vi "Host_Relocation.vi"() -> ()   [LabVIEW 2014]
uses:
  <vilib>/Instr/_visa.llb/VISA Configure Serial Port (Instr).vi
panel:
  out "ERROut?":string
  out "RoughZPrePos":dbl
  in  "Move Forward":bool
  in  "Move Backward":bool
  in  "StepLen um":dbl format="%#_13g"
  in  "MoveTo":bool
  in  "MoveToPos mm":dbl format="%#_13g"
  in  "Confirm":bool
  out "RoughZInitPos mm":dbl
  out "RoughZPosDia":dbl(graph)
  in  "RoughZ":refnum<visa-resource-name>
  out "ERRIn?":string
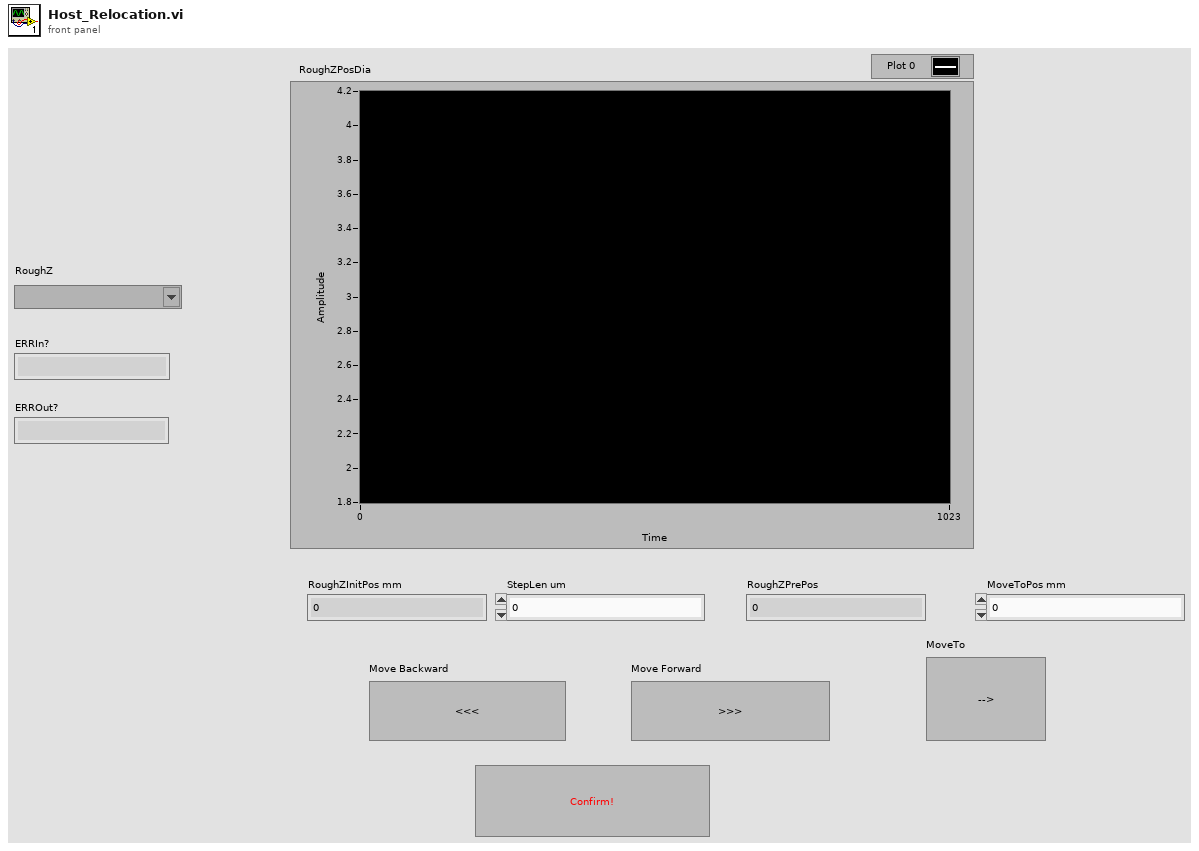
[diagram p1: front panel]
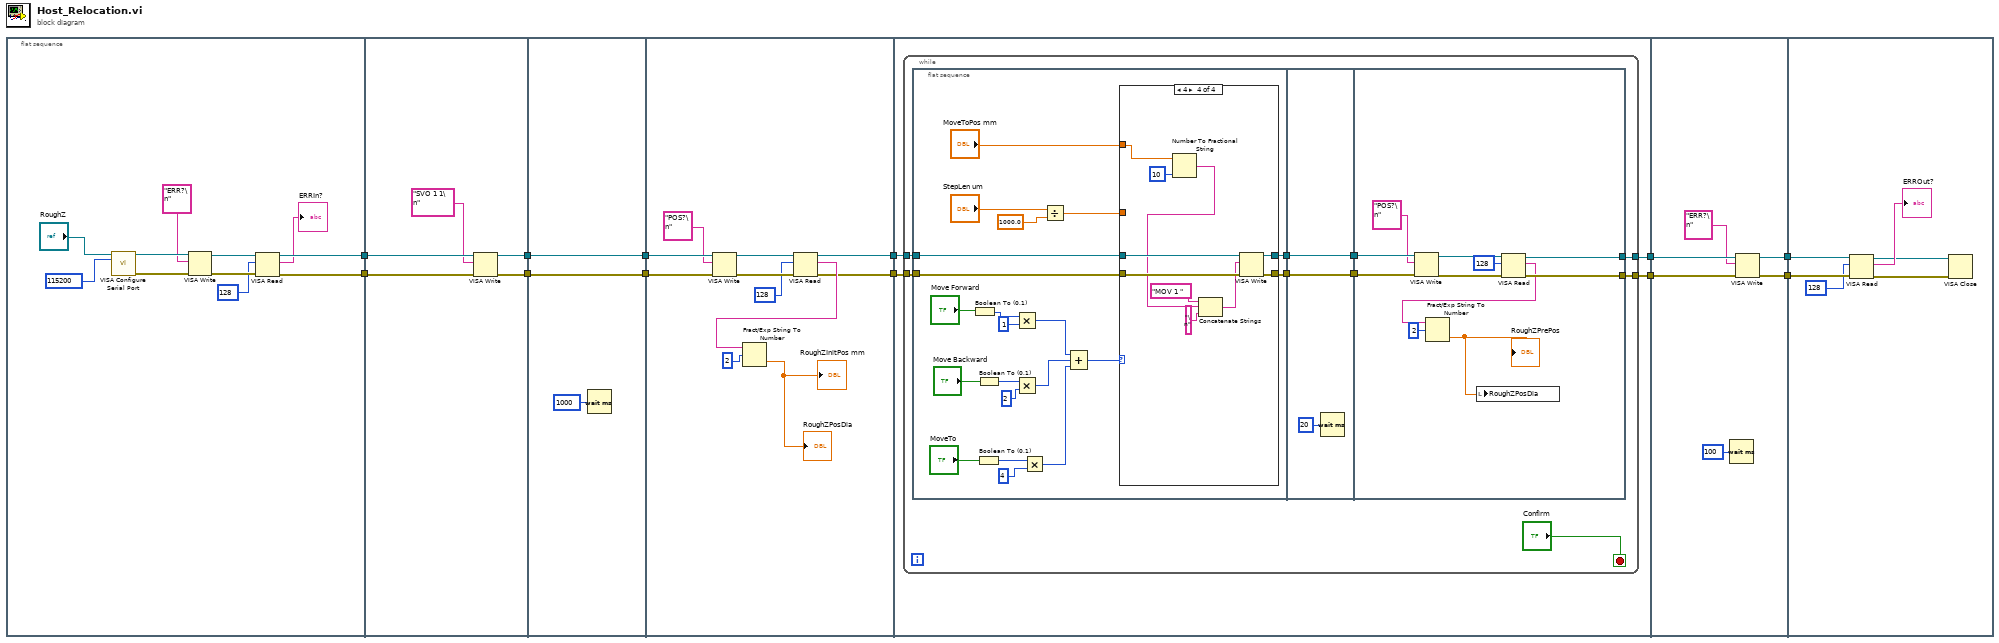
[diagram p0: block diagram]
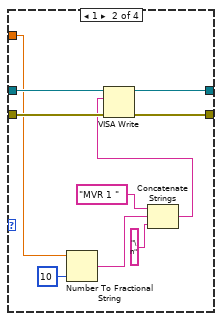
[diagram p3: hidden frame]
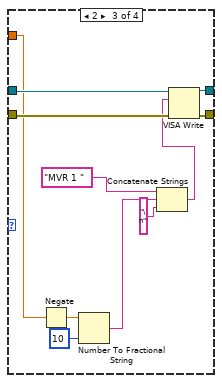
[diagram p4: hidden frame]
diagram:
  n1 = flat-sequence {
    tunnel: [w17] -> w12
    tunnel: [w16] -> w11
    tunnel: w12 -> [w28]
    tunnel: w11 -> [w27]
    tunnel: [w25] -> w10
    tunnel: [w24] -> w9
    tunnel: w10 -> [w30]
    tunnel: w9 -> [w29]
    tunnel: [w30] -> w8
    tunnel: [w29] -> w7
    tunnel: w8 -> [w42]
    tunnel: w7 -> [w41]
    tunnel: [w34] -> w6
    tunnel: [w33] -> w5
    tunnel: w6 -> [w46]
    tunnel: w5 -> [w45]
    tunnel: [w44] -> w4
    tunnel: [w43] -> w3
    tunnel: w4 -> [w128]
    tunnel: w3 -> [w127]
    tunnel: [w125] -> w2
    tunnel: [w124] -> w1
    tunnel: w2 -> [w135]
    tunnel: w1 -> [w134]
    frame #0 {
      n2 = call-poly "VISA Configure Serial Port"("VISA resource name"="RoughZ", "baud rate (9600)"=u32 115200) -> ("VISA resource name out"=w21:refnum<visa-resource-name>, "error out"=w20:errorcluster)  [unwired: 12 in]
      n3 = VISA Write(VISA resource name=w21, write buffer="ERR?\n", error in (no error)=w20) -> (VISA resource name out=w19:refnum<visa-resource-name>, error out=w18:errorcluster)  [unwired: 1 out]
      n4 = VISA Read(VISA resource name=w19, byte count=u32 128, error in (no error)=w18) -> (VISA resource name out=w17:refnum<visa-resource-name>, read buffer=→"ERRIn?":string, error out=w16:errorcluster)  [unwired: 1 out]
    }
    frame #1 {
      n5 = VISA Write(VISA resource name=w28, write buffer="SVO 1 1\n", error in (no error)=w27) -> (VISA resource name out=w25:refnum<visa-resource-name>, error out=w24:errorcluster)  [unwired: 1 out]
    }
    frame #2 {
      n6 = Wait (ms)(milliseconds to wait=u32 1000) -> ()  [unwired: 1 out]
    }
    frame #3 {
      n7 = VISA Write(VISA resource name=w42, write buffer="POS?\n", error in (no error)=w41) -> (VISA resource name out=w39:refnum<visa-resource-name>, error out=w38:errorcluster)  [unwired: 1 out]
      n8 = VISA Read(VISA resource name=w39, byte count=u32 128, error in (no error)=w38) -> (VISA resource name out=w34:refnum<visa-resource-name>, read buffer=w36:string, error out=w33:errorcluster)  [unwired: 1 out]
      n9 = Fract/Exp String To Number(string=w36, offset=2) -> (number=→"RoughZInitPos mm" →"RoughZPosDia":dbl)  [unwired: 2 in, 1 out]
    }
    frame #4 {
      n10 = while {
        tunnel: w46 -> [w54]
        tunnel: w45 -> [w53]
        tunnel: [w48] -> w44
        tunnel: [w47] -> w43
        stop <- "Confirm" stop-if-true
        n11 = flat-sequence {
          tunnel: w54 -> [w67]
          tunnel: w53 -> [w66]
          tunnel: [w65] -> w52
          tunnel: [w64] -> w51
          tunnel: w52 -> [w111]
          tunnel: w51 -> [w110]
          tunnel: [w111] -> w50
          tunnel: [w110] -> w49
          tunnel: w50 -> [w123]
          tunnel: w49 -> [w122]
          tunnel: [w117] -> w48
          tunnel: [w116] -> w47
          frame #0 {
            n12 = Boolean To (0,1)(Boolean="Move Forward") -> (0, 1=w71:i16)
            n13 = Boolean To (0,1)(Boolean="MoveTo") -> (0, 1=w59:i16)
            n14 = Boolean To (0,1)(Boolean="Move Backward") -> (0, 1=w69:i16)
            n15 = Multiply(x=w71, y=i16 1) -> (x*y=w63:i16)
            n16 = Multiply(x=w69, y=i16 2) -> (x*y=w62:i16)
            n17 = Multiply(x=w59, y=i16 4) -> (x*y=w57:i16)
            n18 = Divide(x="StepLen um", y=1000.0) -> (x/y=w74:dbl)
            n19 = Compound Arithmetic op=ADD(w63, w62, w57) -> (w61:i16)
            n20 = case shown="4" w61 {
              tunnel: w74 -> [_ w84 w94 _]
              tunnel: w67 -> [w78 w88 w99 w109]
              tunnel: w66 -> [w77 w87 w98 w108]
              tunnel: [w78 w80 w97 w107] -> w65
              tunnel: [w77 w79 w96 w106] -> w64
              tunnel: "MoveToPos mm" -> [_ _ _ w105]
              frame 0, Default {
              }
              frame 1 {
                n21 = Number To Fractional String(number=w84, precision (6)=i16 10) -> (F-format string=w82:string)  [unwired: 2 in]
                n22 = Concatenate Strings("MVR 1 " ("string"), w82, "\n" ("string")) -> (w86:string)
                n23 = VISA Write(VISA resource name=w88, write buffer=w86, error in (no error)=w87) -> (VISA resource name out=w80:refnum<visa-resource-name>, error out=w79:errorcluster)  [unwired: 1 out]
              }
              frame 2 {
                n24 = Negate(x=w94) -> (-x=w95:dbl)
                n25 = Number To Fractional String(number=w95, precision (6)=i16 10) -> (F-format string=w91:string)  [unwired: 2 in]
                n26 = Concatenate Strings("MVR 1 " ("string"), w91, "\n" ("string")) -> (w89:string)
                n27 = VISA Write(VISA resource name=w99, write buffer=w89, error in (no error)=w98) -> (VISA resource name out=w97:refnum<visa-resource-name>, error out=w96:errorcluster)  [unwired: 1 out]
              }
              frame 4 {
                n28 = Number To Fractional String(number=w105, precision (6)=i16 10) -> (F-format string=w103:string)  [unwired: 2 in]
                n29 = Concatenate Strings("MOV 1 " ("string"), w103, "\n" ("string")) -> (w100:string)
                n30 = VISA Write(VISA resource name=w109, write buffer=w100, error in (no error)=w108) -> (VISA resource name out=w107:refnum<visa-resource-name>, error out=w106:errorcluster)  [unwired: 1 out]
              }
            }
          }
          frame #1 {
            n31 = Wait (ms)(milliseconds to wait=u32 20) -> ()  [unwired: 1 out]
          }
          frame #2 {
            n32 = VISA Write(VISA resource name=w123, write buffer="POS?\n", error in (no error)=w122) -> (VISA resource name out=w121:refnum<visa-resource-name>, error out=w120:errorcluster)  [unwired: 1 out]
            n33 = VISA Read(VISA resource name=w121, byte count=u32 128, error in (no error)=w120) -> (VISA resource name out=w117:refnum<visa-resource-name>, read buffer=w115:string, error out=w116:errorcluster)  [unwired: 1 out]
            n34 = Fract/Exp String To Number(string=w115, offset=2) -> (number=w113:dbl)  [unwired: 2 in, 1 out]
            "RoughZPrePos" <- w113
            n35 = local write "RoughZPosDia"(w113) -> ()
          }
        }
      }
    }
    frame #5 {
      n36 = Wait (ms)(milliseconds to wait=u32 100) -> ()  [unwired: 1 out]
      n37 = VISA Write(VISA resource name=w128, write buffer="ERR?\n", error in (no error)=w127) -> (VISA resource name out=w125:refnum<visa-resource-name>, error out=w124:errorcluster)  [unwired: 1 out]
    }
    frame #6 {
      n38 = VISA Read(VISA resource name=w135, byte count=u32 128, error in (no error)=w134) -> (VISA resource name out=w131:refnum<visa-resource-name>, read buffer=→"ERROut?":string, error out=w130:errorcluster)  [unwired: 1 out]
      n39 = VISA Close(VISA resource name=w131, error in (no error)=w130) -> ()  [unwired: 1 out]
    }
  }
